vi "Read DataObj.vi"(8 "error in (no error)":errorcluster, 11 "Instr Exe Write to File in":refnum<class "Instr Exe Write to File.lvclass">) -> (0 "error out":errorcluster, 2 "DataObj":string, 3 "Instr Exe Write to File out":refnum<class "Instr Exe Write to File.lvclass">)   [LabVIEW 2014, in "Controller.lvlib" / "Instr Exe Write to File.lvclass"]
uses:
  Instr Exe Write to File.lvclass
  Instr Exe Write to File.lvclass/Instr Exe Write to File.ctl
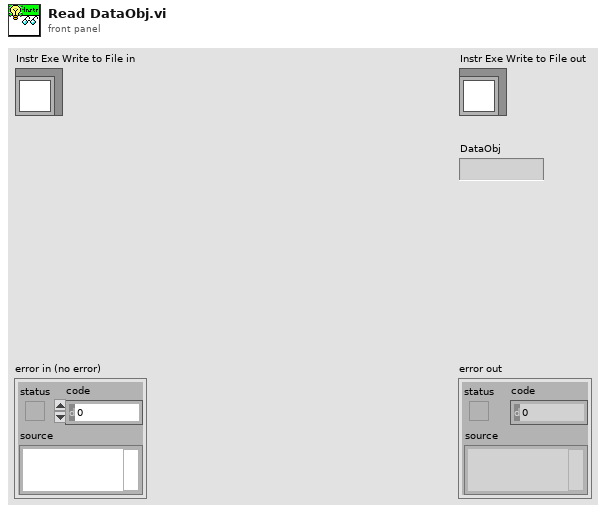
[diagram p1: front panel]
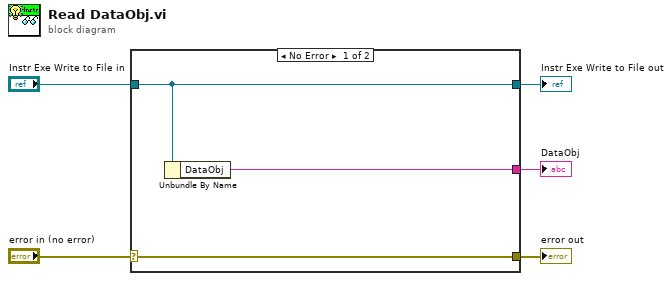
[diagram p0: block diagram]
diagram:
  n1 = case shown="No Error" "error in (no error)" {
    selector: "error in (no error)" -> [w8 w9]
    tunnel: [w8 w9] -> w4
    tunnel: [w7 w10] -> w2
    tunnel: "Instr Exe Write to File in" -> [w7 w10]
    tunnel: [w6 _] -> w1
    frame No Error {
      n2 = Unbundle By Name(w7) -> ("DataObj"=w6:string)
    }
    frame Error {
    }
  }
  "error out" <- w4
  "Instr Exe Write to File out" <- w2
  "DataObj" <- w1
